vi "autodetectPorts.vi"(11 "NXT/EV3":T1) -> ()   [LabVIEW 2013]
uses:
  <vilib>/NXT/Subs/LVHSConnector.ctl
  <vilib>/NXT/LegoClasses/BrickReference/BrickReference.lvclass
  <vilib>/NXT/Dual Mode Library/Advanced/NXTFlag_Assign_integer.vi
  <vilib>/NXT/Dual Mode Library/Advanced/NXTFlag_Get.vi
  <vilib>/NXT/Dual Mode Library/Waits/Wait_Num.vi
  <vilib>/NXT/Dual Mode Library/Advanced/NXTFlag_Get_Integer.vi
  <vilib>/NXT/Dual Mode Library/Motors/Rotation.vi
  <vilib>/NXT/NXTIO Xnodes/NXTIONodeSubVIs/LEGOStopAllMotors.vi
  <vilib>/NXT/NXTIO Xnodes/NXTIOXNode/NXTIO.xnode
  <resource>/objmgr/EV3Primitive.rc
  <vilib>/NXT/Dual Mode Library/Display/drawNumber.vi
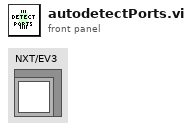
[diagram p1: front panel]
types:
  T1 = typedef "LVHSConnector.ctl" = refnum<class "BrickReference.lvclass">
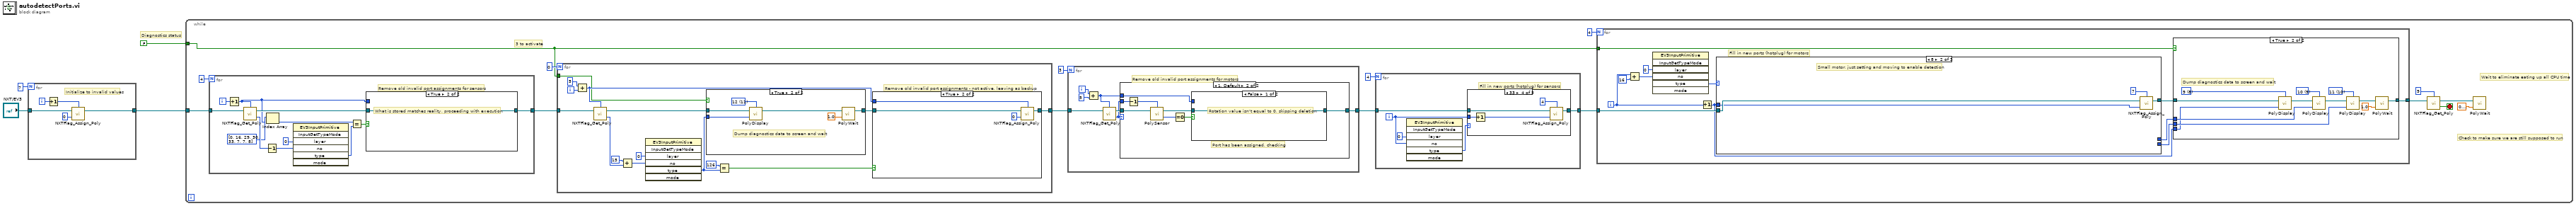
[diagram p0: block diagram]
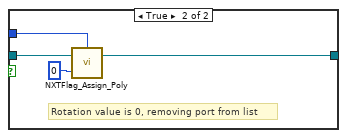
[diagram p3: hidden frame]
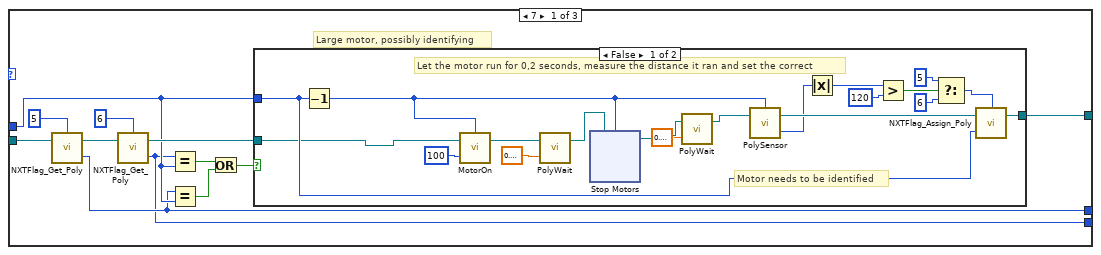
[diagram p7: hidden frame]
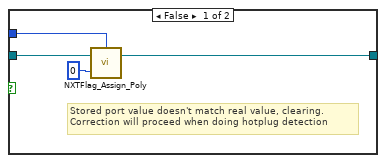
[diagram p10: hidden frame]
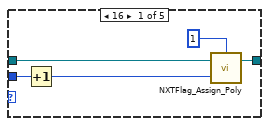
[diagram p11: hidden frame]
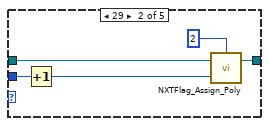
[diagram p12: hidden frame]
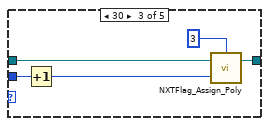
[diagram p13: hidden frame]
diagram:
  # "Diagnostics status"
  n1 = for {
    N: 7 -> [_]
    tunnel: "NXT/EV3" -> [w8]
    tunnel: [w7] -> w2
    i -> [w5]
    # "Initialize to invalid values"
    n2 = Increment(x=w5) -> (x+1=w6:i32)
    n3 = call-poly <vilib>:"NXTFlag_Assign_Poly.vi"("Flag Value"=0, "NXT/EV3"=w8, "NXT/EV3 Flag Number"=w6) -> ("NXT/EV3"=w7:T1)  [unwired: 1 in]
  }
  n4 = while {
    tunnel: w2 -> [w19]
    tunnel: FALSE -> [w10]
    stop <- w21 stop-if-true
    # "3 to activate"
    # "Wait to eliminate eating up all CPU time"
    # "Check to make sure we are still supposed to run"
    n5 = for {
      N: 4 -> [_]
      tunnel: [w144] -> w15
      tunnel: w19 -> [w142]
      i -> [w152]
      # "Remove old invalid port assignments for sensors"
      n6 = Increment(x=w152) -> (x+1=w143:i32)
      n7 = call-poly <vilib>:"NXTFlag_Get_Poly.vi"("NXT/EV3"=w142, "NXT/EV3 Flag Number"=w143) -> ("Flag Value"=w150:i32, "NXT/EV3"=w145:T1)  [unwired: 1 in]
      n8 = Decrement(x=w150) -> (x-1=w141:i32)
      n9 = Index Array(array=i32[] [0, 16, 29, 30, 33, 7, 7, 8], index=w143) -> (element=w147:i32)
      n10 = invoke class="EV3InputPrimitive" method="InputGetTypeMode"("layer"=u8 0, "no"=w141) -> ("type"=w148:u8)  [unwired: 5 in, 6 out]
      n11 = Equal?(x=w147, y=w148) -> (x = y?=w146:bool)
      n12 = case shown="True" w146 {
        tunnel: [w156 w157] -> w144
        tunnel: w145 -> [w155 w157]
        tunnel: w143 -> [w153 _]
        frame False {
          # "Stored port value doesn't match real value, clearing.\nCorrection will proceed when doing hotplug detection"
          n13 = call-poly <vilib>:"NXTFlag_Assign_Poly.vi"("Flag Value"=0, "NXT/EV3"=w155, "NXT/EV3 Flag Number"=w153) -> ("NXT/EV3"=w156:T1)  [unwired: 1 in]
        }
        frame True {
          # "What is stored matches reality, proceeding with execution"
        }
      }
    }
    n14 = for {
      N: 0 -> [_]
      tunnel: [w47] -> w13
      tunnel: w15 -> [w55]
      tunnel: w10 -> [w48]
      i -> [w61]
      # "Remove old invalid port assignments - not active, leaving as backup"
      n15 = Add(x=5, y=w61) -> (x+y=w56:i32)
      n16 = call-poly <vilib>:"NXTFlag_Get_Poly.vi"("NXT/EV3"=w55, "NXT/EV3 Flag Number"=w56) -> ("Flag Value"=w59:i32, "NXT/EV3"=w57:T1)  [unwired: 1 in]
      n17 = Add(x=15, y=w59) -> (x+y=w54:i32)
      n18 = invoke class="EV3InputPrimitive" method="InputGetTypeMode"("layer"=u8 0, "no"=w54) -> ("type"=w49:u8)  [unwired: 5 in, 6 out]
      n19 = case shown="True" w48 {
        tunnel: w57 -> [w62 w68]
        tunnel: [w62 w63] -> w50
        tunnel: w49 -> [_ w66]
        frame False {
        }
        frame True {
          w67 = i16 11 items=["1", "2", "3", "4", "5", "6", "7", "8", "9", "10", "11", "12"] ("Line")
          # "Dump diagnostics data to screen and wait"
          n20 = call-poly <vilib>:"PolyDisplay.vi"("number"=w66, "NXT/EV3"=w68, "Line"=w67) -> ("NXT/EV3"=w64:T1)  [unwired: 1 in]
          n21 = call-poly <vilib>:"PolyWait.vi"("Time (1 sec)"=sgl 1.0, "NXT/EV3"=w64) -> ("NXT/EV3"=w63:T1)  [unwired: 2 in]
        }
      }
      n22 = Equal?(x=u8 126, y=w49) -> (x = y?=w58:bool)
      n23 = case shown="True" w58 {
        tunnel: [w69 w73] -> w47
        tunnel: w50 -> [w69 w72]
        tunnel: w56 -> [_ w70]
        frame False {
        }
        frame True {
          n24 = call-poly <vilib>:"NXTFlag_Assign_Poly.vi"("Flag Value"=0, "NXT/EV3"=w72, "NXT/EV3 Flag Number"=w70) -> ("NXT/EV3"=w73:T1)  [unwired: 1 in]
        }
      }
    }
    n25 = for {
      N: 3 -> [_]
      tunnel: [w30] -> w12
      tunnel: w13 -> [w32]
      i -> [w29]
      # "Remove old invalid port assignments for motors"
      n26 = Add(x=w29, y=5) -> (x+y=w26:i32)
      n27 = call-poly <vilib>:"NXTFlag_Get_Poly.vi"("NXT/EV3"=w32, "NXT/EV3 Flag Number"=w26) -> ("Flag Value"=w27:i32, "NXT/EV3"=w31:T1)  [unwired: 1 in]
      n28 = case shown="1, Default" w27 {
        tunnel: w31 -> [w33 w41]
        tunnel: [w33 w38] -> w30
        tunnel: w27 -> [_ w39]
        tunnel: w26 -> [_ w36]
        frame 0 {
          # "Port never assigned or already cleared"
        }
        frame 1, Default {
          # "Port has been assigned, checking"
          n29 = Decrement(x=w39) -> (x-1=w40:i32)
          n30 = call-poly <vilib>:"PolySensor.vi"("NXT/EV3"=w41, "Port (Port A)"=w40) -> ("Angle of Rotation"=w35:i32, "NXT/EV3"=w37:T1)  [unwired: 1 in]
          n31 = Equal To 0?(x=w35) -> (x = 0?=w34:bool)
          n32 = case shown="False" w34 {
            tunnel: [w42 w46] -> w38
            tunnel: w37 -> [w42 w45]
            tunnel: w36 -> [_ w43]
            frame False {
              # "Rotation value isn't equal to 0, skipping deletion"
            }
            frame True {
              # "Rotation value is 0, removing port from list"
              n33 = call-poly <vilib>:"NXTFlag_Assign_Poly.vi"("Flag Value"=0, "NXT/EV3"=w45, "NXT/EV3 Flag Number"=w43) -> ("NXT/EV3"=w46:T1)  [unwired: 1 in]
            }
          }
        }
      }
    }
    n34 = for {
      N: 4 -> [_]
      tunnel: [w160] -> w18
      tunnel: w12 -> [w158]
      i -> [w159]
      # "Fill in new ports (hotplug) for sensors"
      n35 = invoke class="EV3InputPrimitive" method="InputGetTypeMode"("layer"=u8 0, "no"=w159) -> ("type"=w161:u8)  [unwired: 5 in, 6 out]
      n36 = case shown="33" w161 {
        tunnel: [w166 w169 w177 w181 w183] -> w160
        tunnel: w159 -> [w164 w170 w175 w180 _]
        tunnel: w158 -> [w163 w168 w173 w178 w183]
        frame 16 {
          n37 = Increment(x=w164) -> (x+1=w165:i32)
          n38 = call-poly <vilib>:"NXTFlag_Assign_Poly.vi"("Flag Value"=w165, "NXT/EV3"=w163, "NXT/EV3 Flag Number"=i8 1) -> ("NXT/EV3"=w166:T1)  [unwired: 1 in]
        }
        frame 29 {
          n39 = Increment(x=w170) -> (x+1=w171:i32)
          n40 = call-poly <vilib>:"NXTFlag_Assign_Poly.vi"("Flag Value"=w171, "NXT/EV3"=w168, "NXT/EV3 Flag Number"=i8 2) -> ("NXT/EV3"=w169:T1)  [unwired: 1 in]
        }
        frame 30 {
          n41 = Increment(x=w175) -> (x+1=w174:i32)
          n42 = call-poly <vilib>:"NXTFlag_Assign_Poly.vi"("Flag Value"=w174, "NXT/EV3"=w173, "NXT/EV3 Flag Number"=i8 3) -> ("NXT/EV3"=w177:T1)  [unwired: 1 in]
        }
        frame 33 {
          n43 = Increment(x=w180) -> (x+1=w179:i32)
          n44 = call-poly <vilib>:"NXTFlag_Assign_Poly.vi"("Flag Value"=w179, "NXT/EV3"=w178, "NXT/EV3 Flag Number"=i8 4) -> ("NXT/EV3"=w181:T1)  [unwired: 1 in]
        }
        frame 126, Default {
          # "Port is unwired, do nothing"
        }
      }
    }
    n45 = for {
      N: 4 -> [_]
      tunnel: [w80] -> w17
      tunnel: w18 -> [w83]
      tunnel: w10 -> [w74]
      i -> [w78]
      # "Fill in new ports (hotplug) for motors"
      n46 = Add(x=w78, y=16) -> (x+y=w82:i32)
      n47 = invoke class="EV3InputPrimitive" method="InputGetTypeMode"("layer"=u8 0, "no"=w82) -> ("type"=w79:u8)  [unwired: 5 in, 6 out]
      n48 = Increment(x=w78) -> (x+1=w75:i32)
      n49 = case shown="8" w79 {
        tunnel: [w110 w138 w140] -> w84
        tunnel: w75 -> [w101 w136 _]
        tunnel: w83 -> [w109 w139 w140]
        tunnel: [w100 _ _] -> w77
        tunnel: [w99 _ _] -> w76
        frame 7 {
          # "Large motor, possibly identifying"
          n50 = call-poly <vilib>:"NXTFlag_Get_Poly.vi"("NXT/EV3"=w109, "NXT/EV3 Flag Number"=5) -> ("Flag Value"=w100:i32, "NXT/EV3"=w107:T1)  [unwired: 1 in]
          n51 = call-poly <vilib>:"NXTFlag_Get_Poly.vi"("NXT/EV3"=w107, "NXT/EV3 Flag Number"=6) -> ("Flag Value"=w99:i32, "NXT/EV3"=w106:T1)  [unwired: 1 in]
          n52 = Equal?(x=w99, y=w101) -> (x = y?=w104:bool)
          n53 = Equal?(x=w100, y=w101) -> (x = y?=w103:bool)
          n54 = Or(x=w104, y=w103) -> (x .or. y?=w102:bool)
          n55 = case shown="False" w102 {
            tunnel: [w129 w135] -> w110
            tunnel: w106 -> [w111 w135]
            tunnel: w101 -> [w116 _]
            frame False {
              # "Let the motor run for 0,2 seconds, measure the distance it ran and set the correct"
              # "Motor needs to be identified"
              n56 = Decrement(x=w116) -> (x-1=w115:i32)
              n57 = call <vilib>:"MotorOn.vi"("Power (75)"=100, "NXT/EV3"=w111, "Output Port (All Ports)"=w115) -> ("NXT/EV3"=w124:T1)  [unwired: 1 in]
              n58 = call-poly <vilib>:"PolyWait.vi"("Time (1 sec)"=sgl 0.2, "NXT/EV3"=w124) -> ("NXT/EV3"=w122:T1)  [unwired: 2 in]
              n59 = xnode "Stop Motors"("Motors"=w115, "NXT/EV3"=w122) -> ("NXT/EV3"=w114:T1)
              n60 = call-poly <vilib>:"PolyWait.vi"("Time (1 sec)"=sgl 0.1, "NXT/EV3"=w114) -> ("NXT/EV3"=w112:T1)  [unwired: 2 in]
              n61 = call-poly <vilib>:"PolySensor.vi"("NXT/EV3"=w112, "Port (Port A)"=w115) -> ("Angle of Rotation"=w120:i32, "NXT/EV3"=w121:T1)  [unwired: 1 in]
              n62 = Absolute Value(x=w120) -> (abs(x)=w119:i32)
              n63 = Greater?(x=w119, y=120) -> (0:w117:bool)
              n64 = Select(t=5, s=w117, f=6) -> (s? t:f=w128:i32)
              n65 = call-poly <vilib>:"NXTFlag_Assign_Poly.vi"("Flag Value"=w116, "NXT/EV3"=w121, "NXT/EV3 Flag Number"=w128) -> ("NXT/EV3"=w129:T1)  [unwired: 1 in]
            }
            frame True {
              # "Already know this motor, skipping identification"
            }
          }
        }
        frame 8 {
          # "Small motor, just setting and moving to enable detection"
          n66 = call-poly <vilib>:"NXTFlag_Assign_Poly.vi"("Flag Value"=w136, "NXT/EV3"=w139, "NXT/EV3 Flag Number"=i8 7) -> ("NXT/EV3"=w138:T1)  [unwired: 1 in]
        }
        frame 126, Default {
          # "Port is unwired, do nothing"
        }
      }
      n67 = case shown="True" w74 {
        tunnel: w84 -> [w86 w88]
        tunnel: [w86 w89] -> w80
        tunnel: w77 -> [_ w93]
        tunnel: w76 -> [_ w92]
        tunnel: w75 -> [_ w91]
        frame False {
        }
        frame True {
          w94 = i16 10 items=["1", "2", "3", "4", "5", "6", "7", "8", "9", "10", "11", "12"] ("Line")
          w95 = i16 9 items=["1", "2", "3", "4", "5", "6", "7", "8", "9", "10", "11", "12"] ("Line")
          w96 = i16 8 items=["1", "2", "3", "4", "5", "6", "7", "8", "9", "10", "11", "12"] ("Line")
          # "Dump diagnostics data to screen and wait"
          n68 = call-poly <vilib>:"PolyDisplay.vi"("number"=w91, "NXT/EV3"=w88, "Line"=w96) -> ("NXT/EV3"=w98:T1)  [unwired: 1 in]
          n69 = call-poly <vilib>:"PolyDisplay.vi"("number"=w93, "NXT/EV3"=w98, "Line"=w95) -> ("NXT/EV3"=w97:T1)  [unwired: 1 in]
          n70 = call-poly <vilib>:"PolyDisplay.vi"("number"=w92, "NXT/EV3"=w97, "Line"=w94) -> ("NXT/EV3"=w90:T1)  [unwired: 1 in]
          n71 = call-poly <vilib>:"PolyWait.vi"("Time (1 sec)"=sgl 1.0, "NXT/EV3"=w90) -> ("NXT/EV3"=w89:T1)  [unwired: 2 in]
        }
      }
    }
    n72 = call-poly <vilib>:"NXTFlag_Get_Poly.vi"("NXT/EV3"=w17, "NXT/EV3 Flag Number"=9) -> ("status"=w21:bool, "NXT/EV3"=w22:T1)  [unwired: 1 in]
    n73 = call-poly <vilib>:"PolyWait.vi"("Time (1 sec)"=sgl 0.1, "NXT/EV3"=w22) -> ()  [unwired: 2 in, 1 out]
  }
